vi "Clock State Machine.vi"(0 "Boolean in":bool) -> (8 "Boolean out":bool)   [LabVIEW 2011]
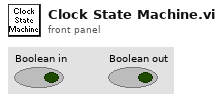
[diagram p1: front panel]
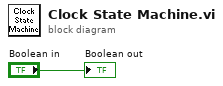
[diagram p0: block diagram]
diagram:
  "Boolean out" <- "Boolean in"
